vi "Array Test.vi"() -> ()   [LabVIEW 2021]
panel:
  out "min index(es)":i32[](array[numeric])
  out "min value":dbl
  out "max index(es)":i32[](array[numeric])
  out "max value":dbl
  out "Array":dbl[][](array[numeric])
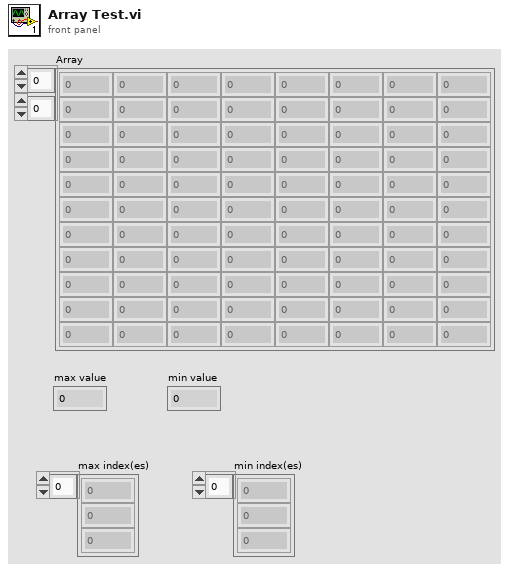
[diagram p1: front panel]
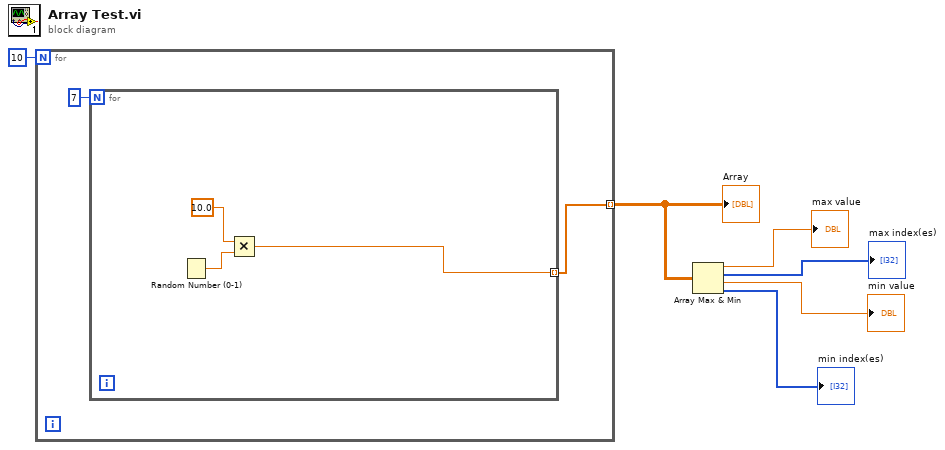
[diagram p0: block diagram]
diagram:
  n1 = for {
    N: 10 -> [_]
    tunnel: [w8] -> w6 mode=indexing
    n2 = for {
      N: 7 -> [_]
      tunnel: [w9] -> w8 mode=indexing
      n3 = Random Number (0-1)() -> (number: 0 to 1=w11:dbl)
      n4 = Multiply(x=10.0, y=w11) -> (x*y=w9:dbl)
    }
  }
  "Array" <- w6
  n5 = Array Max & Min(array=w6) -> (max value=→"max value":dbl, max index (indices)=→"max index(es)":i32[], min value=→"min value":dbl, min index (indices)=→"min index(es)":i32[])
